vi "cfg editor.vi"() -> ()   [LabVIEW 2010]
panel:
  in  "Tab Control":enum32{"_testStepCfg", "paraCfg"}(tab)=enum."paraCfg"
  in  "Test Step CFG EDIT":string[][](table)
  in  "Library function":string(tree)="sigDirMulStatInSet"
  in  "Parameter CFG EDIT":string[][](table)
  in  "para section":string(tree)="parameter section"
  out "View row details":string[](array[string])
  out "error out":errorcluster
  in  "error in":errorcluster
  in  "stop":bool
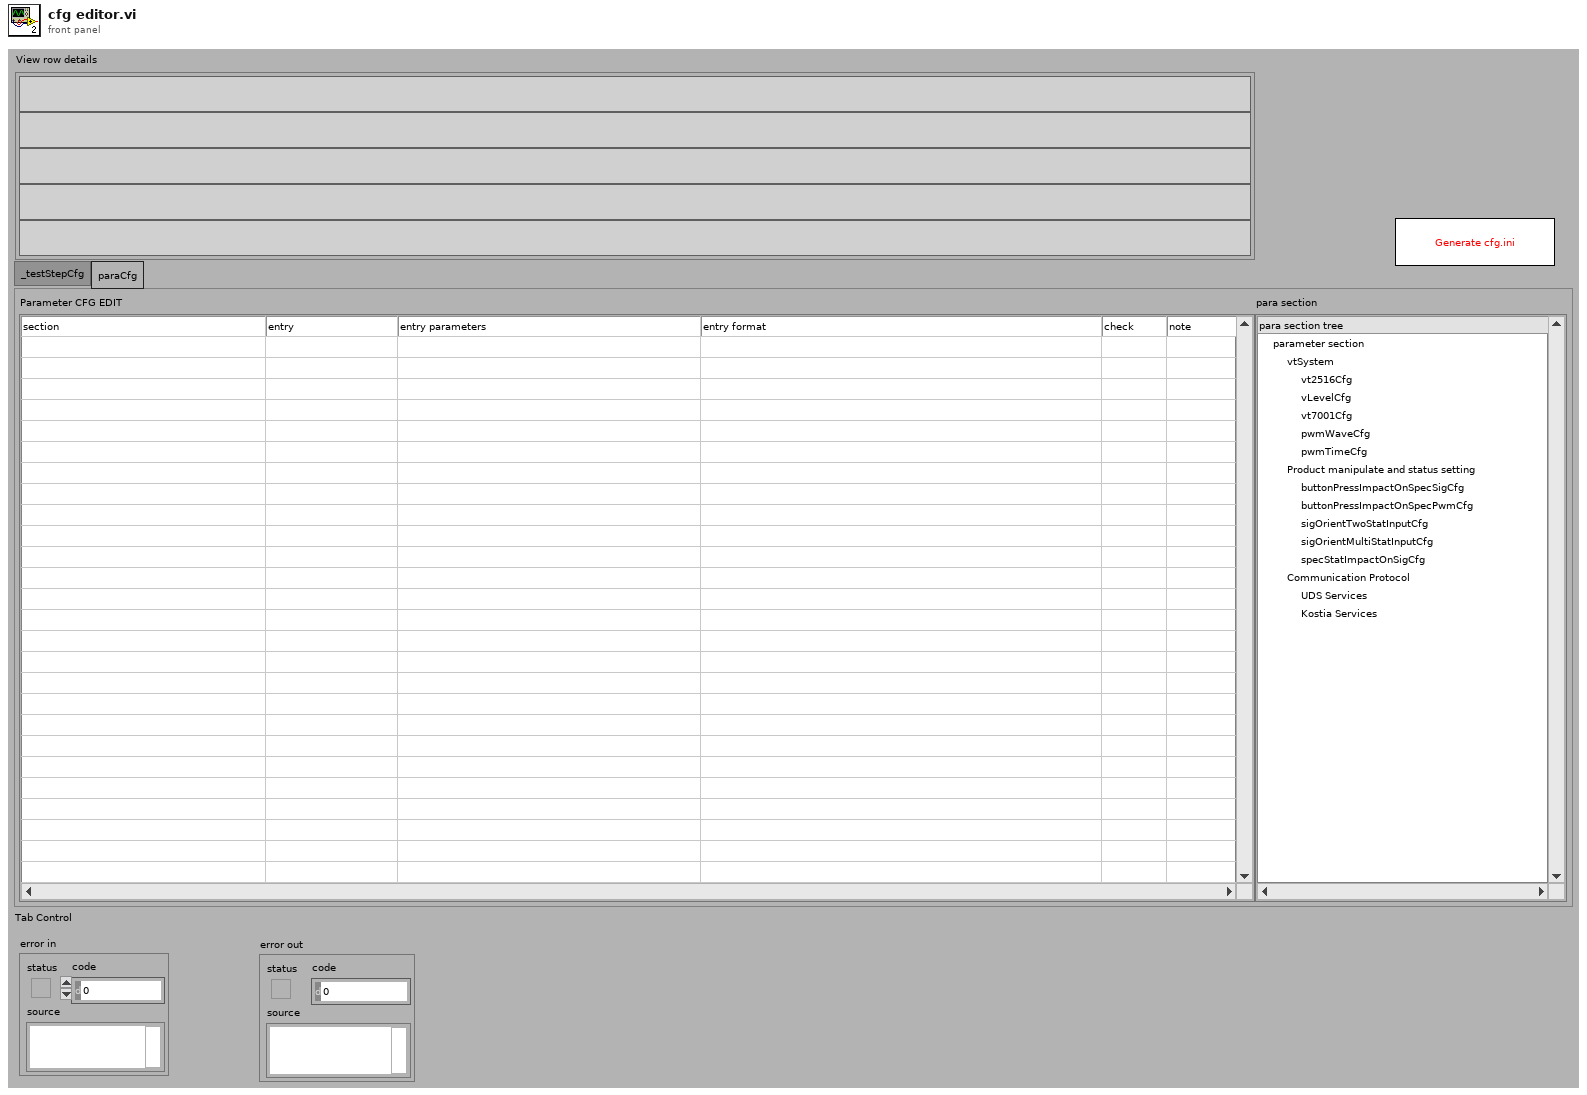
[diagram p1: front panel]
types:
  T1 = typedef "LVRowAndColumnTypeDef.ctl" = cluster{"Row":i32, "Column":i32}
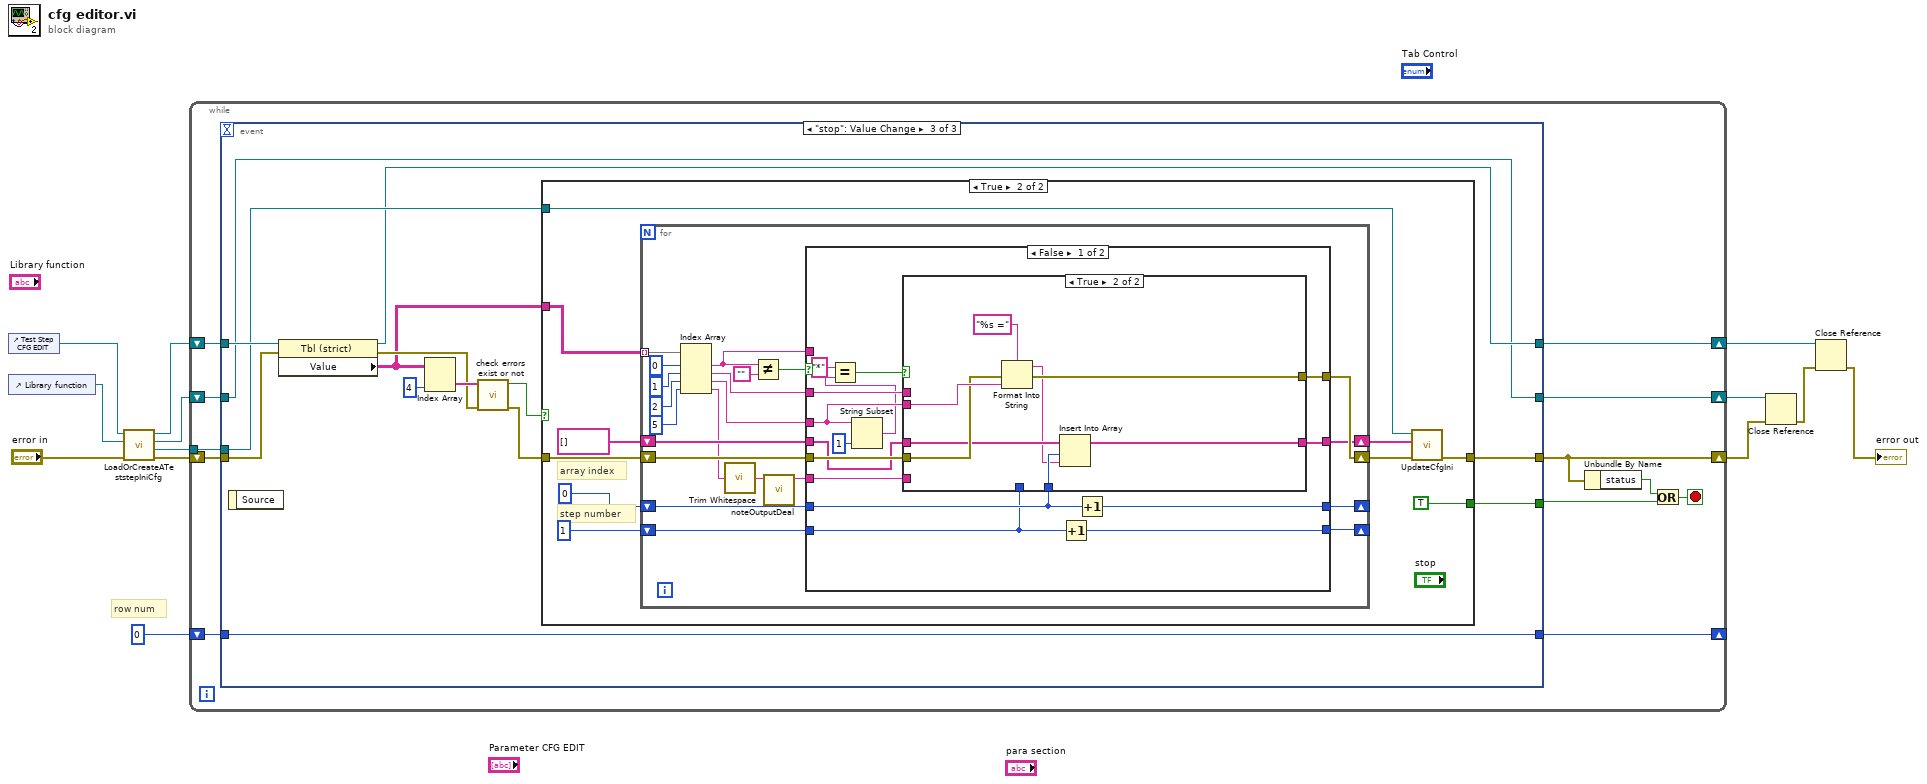
[diagram p0: block diagram]
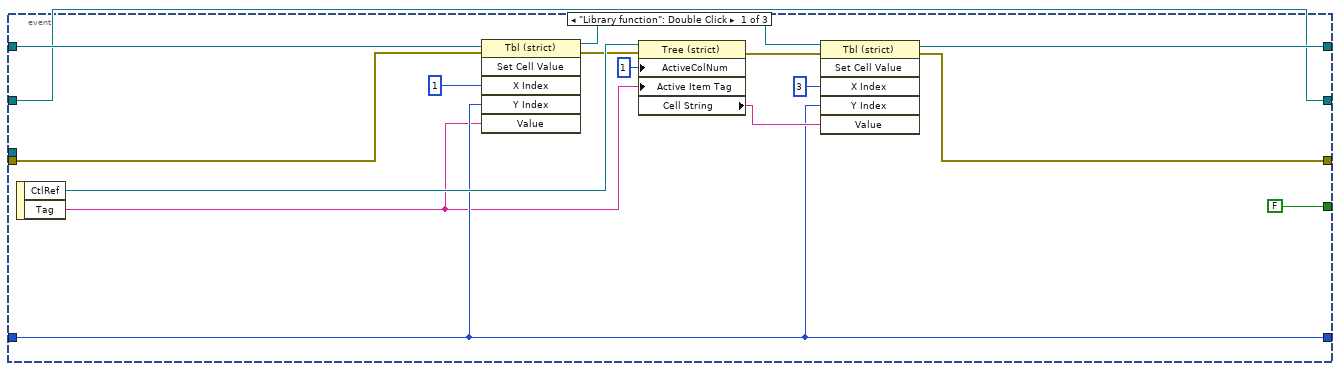
[diagram p2: hidden frame]
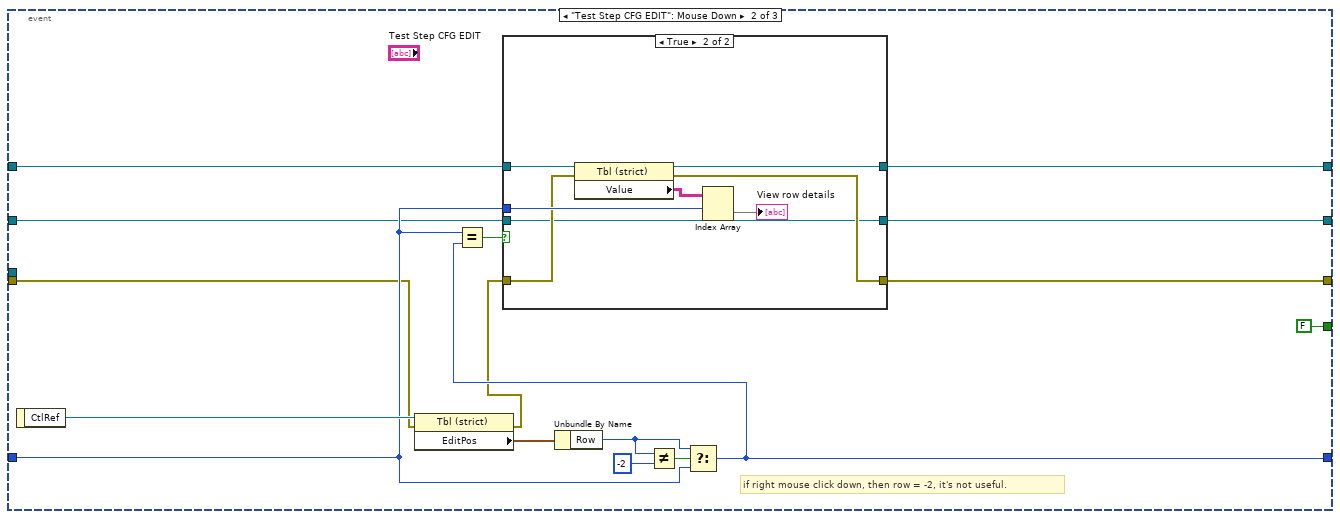
[diagram p3: hidden frame]
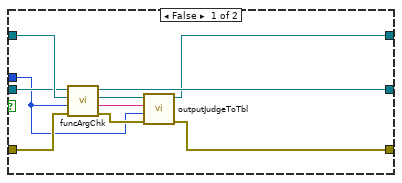
[diagram p4: hidden frame]
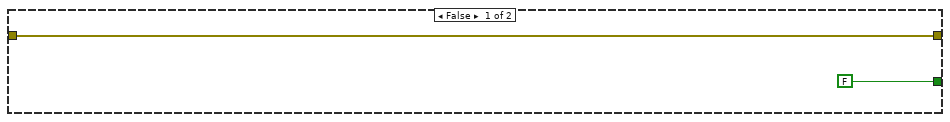
[diagram p5: hidden frame]
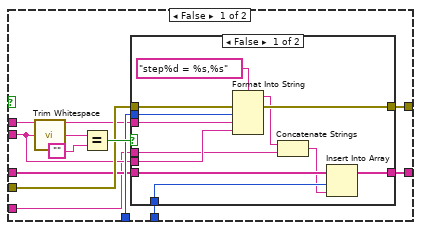
[diagram p6: hidden frame]
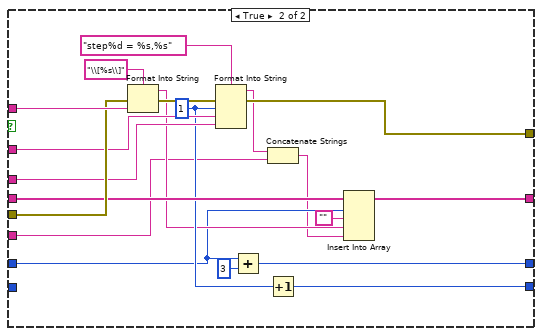
[diagram p8: hidden frame]
diagram:
  # "row num"
  n1 = control-ref of="Test Step CFG EDIT"() -> (w12:refnum<vi>)
  n2 = control-ref of="Library function"() -> (w13:refnum<vi>)
  n3 = call "LoadOrCreateATeststepIniCfg.vi"("error in"="error in", "Tree Refnum"=w13, "Tbl Refnum in"=w12) -> ("error out"=w6:errorcluster, "cfg file refnum out"=w10:refnum<file>, "Tree Refnum out"=w5:refnum<vi>, "Tbl Refnum out"=w7:refnum<vi>)  [unwired: 5 in]
  n4 = while {
    shift-right: [w22] -> w3
    shift-left: w6 -> [w25]
    shift-right: [w18] -> _
    shift-left: 0 ("Row") -> [w19]
    shift-right: [w17] -> w9
    shift-left: w7 -> [w20]
    tunnel: w10 -> [w16]
    shift-right: [w14] -> w4
    shift-left: w5 -> [w15]
    stop <- w23 stop-if-true
    n5 = event shown="[2] \"stop\": Value Change" {
      selector: _ -> [_ _ _]
      dyn-events: _ -> [_ _ _]
      timeout: _ -> [_ _ _]
      tunnel: w25 -> [w40 w45 w85]
      tunnel: [w31 w51 w86] -> w22
      tunnel: [FALSE ("stop") FALSE ("stop") w89] -> w24
      tunnel: w20 -> [w41 w52 w87]
      tunnel: w19 -> [w29 w47 w88]
      tunnel: [w29 w49 w88] -> w18
      tunnel: [w28 w48 w80] -> w17
      tunnel: w16 -> [_ _ w84]
      tunnel: w15 -> [w27 w43 w76]
      tunnel: [w27 w42 w76] -> w14
      event "Library function": Double Click {
        n6 = event-data() -> ("CtlRef"=w38:refnum<vi>, "Tag"=w26:string)  [unwired: 1 in]
        n7 = invoke class="Tbl (strict)" method="Set Cell Value"(reference=w41, error in=w40, "X Index"=u32 1 ("Y Index"), "Y Index"=w29, "Value"=w26) -> (reference out=w32:refnum<vi>, error out=w33:errorcluster)  [unwired: 1 in, 4 out]
        n8 = property class="Tree (strict)"(reference=w38, error in=w33, "ActiveColNum"=1 ("Active Cell:Active Column Number"), "Active Item Tag"=w26) -> (error out=w36:errorcluster, "Cell String"=w35:string)  [unwired: 1 out]
        n9 = invoke class="Tbl (strict)" method="Set Cell Value"(reference=w32, error in=w36, "X Index"=u32 3, "Y Index"=w29, "Value"=w35) -> (reference out=w28:refnum<vi>, error out=w31:errorcluster)  [unwired: 1 in, 4 out]
      }
      event "Test Step CFG EDIT": Mouse Down {
        # "if right mouse click down, then row = -2, it's not useful."
        n10 = event-data() -> ("CtlRef"=w57:refnum<vi>)  [unwired: 1 in]
        n11 = property class="Tbl (strict)"(reference=w57, error in=w45) -> (error out=w44:errorcluster, "EditPos"=w56:T1)  [unwired: 1 out]
        n12 = Unbundle By Name(w56) -> ("Row"=w53:i32)
        n13 = Not Equal?(x=w53, y=-2) -> (x != y?=w54:bool)
        n14 = Select(t=w53, s=w54, f=w47) -> (s? t:f=w49:i32)
        n15 = Equal?(x=w47, y=w49) -> (x = y?=w50:bool)
        n16 = case shown="True" w50 {
          tunnel: w47 -> [w61 w75]
          tunnel: w52 -> [w66 w73]
          tunnel: w44 -> [w67 w71]
          tunnel: [w58 w70] -> w51
          tunnel: [w59 w69] -> w48
          tunnel: w43 -> [w65 w68]
          tunnel: [w64 w68] -> w42
          frame False {
            n17 = call "funcArgChk.vi"("error in"=w67, "Row number"=w61, "Tbl Refnum in"=w66, "Tree Refnum in"=w65) -> ("error out"=w62:errorcluster, "Check result"=w63:string, "Tbl Refnum out"=w60:refnum<vi>, "Tree Refnum out"=w64:refnum<vi>)  [unwired: 4 in]
            n18 = call "outputJudgeToTbl.vi"("error in"=w62, "rowNum"=w61, "judgeRes"=w63, "Tbl Refnum in"=w60) -> ("error out"=w58:errorcluster, "Tbl Refnum Out"=w59:refnum<vi>)  [unwired: 6 in]
          }
          frame True {
            n19 = property class="Tbl (strict)"(reference=w73, error in=w71) -> (reference out=w69:refnum<vi>, error out=w70:errorcluster, "Value"=w72:string[][])
            n20 = Index Array(array=w72, index (row)=w75) -> (element=→"View row details":string[])  [unwired: 1 in]
          }
        }
      }
      event "stop": Value Change {
        n21 = event-data() -> ()  [unwired: 1 in, 1 out]
        n22 = property class="Tbl (strict)"(reference=w87, error in=w85) -> (reference out=w80:refnum<vi>, error out=w81:errorcluster, "Value"=w77:string[][])
        n23 = Index Array(array=w77, index (col)=4 ("disabled index (col)")) -> (element=w82:string[])  [unwired: 1 in]
        n24 = call "check errors exist or not.vi"("error in"=w81, "judge column"=w82) -> ("error out"=w79:errorcluster, "Go on?"=w78:bool)  [unwired: 8 in]
        n25 = case shown="True" w78 {
          tunnel: [FALSE ("stop") TRUE ("stop")] -> w89
          tunnel: [w90 w92] -> w86
          tunnel: w84 -> [_ w93]
          tunnel: w79 -> [w90 w97]
          tunnel: w77 -> [_ w96]
          frame False {
          }
          frame True {
            # "step number"
            # "array index"
            n26 = for {
              tunnel: w96 -> [w120] mode=indexing
              shift-right: [w110] -> w94
              shift-left: string[] [] ("Value") -> [w114]
              shift-right: [w111] -> w95
              shift-left: w97 -> [w115]
              shift-right: [w109] -> _
              shift-left: 0 ("input 1") -> [w108]
              shift-right: [w107] -> _
              shift-left: 1 ("input 1") -> [w106]
              n27 = Index Array(array=w120, index #1=0 ("index"), index #2=1 ("index"), index #3=2 ("index"), index #4=5 ("index")) -> (element #1=w116:string, element #2=w113:string, element #3=w112:string, element #4=w104:string)
              n28 = call <vilib>:"Trim Whitespace.vi"("string"=w104) -> ("trimmed string"=w103:string)  [unwired: 1 in]
              n29 = Not Equal?(x=w116, y="") -> (x != y?=w117:bool)
              n30 = call "noteOutputDeal.vi"("note in editor"=w103) -> ("note output"=w102:string)  [unwired: 10 in]
              n31 = case shown="False" w117 {
                tunnel: w116 -> [_ w190]
                tunnel: w115 -> [w137 w189]
                tunnel: w114 -> [w126 w188]
                tunnel: w113 -> [w128 w185]
                tunnel: w112 -> [w127 w184]
                tunnel: [w136 w183] -> w111
                tunnel: [w125 w182] -> w110
                tunnel: [w135 w176] -> w109
                tunnel: w108 -> [w134 w175]
                tunnel: [w132 w180] -> w107
                tunnel: w106 -> [w133 _]
                tunnel: w102 -> [w123 w173]
                frame False {
                  n32 = String Subset(string=w127, length (rest)=1 ("length (rest)")) -> (substring=w124:string)  [unwired: 1 in]
                  n33 = Equal?(x="*", y=w124) -> (x = y?=w130:bool)
                  n34 = case shown="True" w130 {
                    tunnel: w137 -> [w145 w169]
                    tunnel: [w139 w168] -> w136
                    tunnel: w134 -> [w142 w167]
                    tunnel: w133 -> [w146 _]
                    tunnel: w128 -> [w144 _]
                    tunnel: w127 -> [w143 w170]
                    tunnel: w126 -> [w141 w166]
                    tunnel: [w140 w165] -> w125
                    tunnel: w123 -> [w138 _]
                    frame False {
                      n35 = call <vilib>:"Trim Whitespace.vi"("string"=w143) -> ("trimmed string"=w149:string)  [unwired: 1 in]
                      n36 = Equal?(x=w149, y="") -> (x = y?=w147:bool)
                      n37 = case shown="False" w147 {
                        tunnel: w146 -> [w160 _]
                        tunnel: w145 -> [w159 w162]
                        tunnel: w144 -> [w158 _]
                        tunnel: w143 -> [w157 _]
                        tunnel: w142 -> [w156 _]
                        tunnel: w141 -> [w155 w163]
                        tunnel: [w154 w163] -> w140
                        tunnel: [w153 w162] -> w139
                        tunnel: w138 -> [w151 _]
                        frame False {
                          n38 = Format Into String(format string="step%d = %s,%s", error in=w159, w160, w158, w157) -> (resulting string=w152:string, error out=w153:errorcluster)  [unwired: 1 in]
                          n39 = Concatenate Strings(w152, w151) -> (w150:string)
                          n40 = Insert Into Array(array=w155, index=w156, new element=w150) -> (w154:string[])
                        }
                        frame True {
                        }
                      }
                    }
                    frame True {
                      n41 = Format Into String(format string="%s =", error in=w169, w170) -> (resulting string=w164:string, error out=w168:errorcluster)  [unwired: 1 in]
                      n42 = Insert Into Array(array=w166, index=w167, new element=w164) -> (w165:string[])
                    }
                  }
                  n43 = Increment(x=w133) -> (x+1=w132:i32)
                  n44 = Increment(x=w134) -> (x+1=w135:i32)
                }
                frame True {
                  w181 = 1 ("input 1")
                  n45 = Format Into String(format string="\\[%s\\]", error in=w189, w190) -> (resulting string=w179:string, error out=w186:errorcluster)  [unwired: 1 in]
                  n46 = Format Into String(format string="step%d = %s,%s", error in=w186, w181, w185, w184) -> (resulting string=w174:string, error out=w183:errorcluster)  [unwired: 1 in]
                  n47 = Add(x=w175, y=3) -> (x+y=w176:i32)
                  n48 = Concatenate Strings(w174, w173) -> (w172:string)
                  n49 = Increment(x=w181) -> (x+1=w180:i32)
                  n50 = Insert Into Array(array=w188, index=w175, new element #1="", new element #2=w179, new element #3=w172) -> (w182:string[])
                }
              }
            }
            n51 = call "UpdateCfgIni.vi"("error in"=w95, "contentArray"=w94, "iniCfgRefnumIn"=w93) -> ("error out"=w92:errorcluster)  [unwired: 8 in]
          }
        }
      }
    }
    n52 = Unbundle By Name(w22) -> ("status"=w21:bool)
    n53 = Or(x=w21, y=w24) -> (x .or. y?=w23:bool)
  }
  n54 = Close Reference(reference=w4, error in (no error)=w3) -> (error out=w2:errorcluster)
  n55 = Close Reference(reference=w9, error in (no error)=w2) -> (error out=→"error out":errorcluster)
